vi "Link_Call Unlink.vi"(8 "error in (no error)":errorcluster, 11 "Run Data in":T1={"Target Folder"=path "", "Menu Folder"=path "", "Active Folder"=path "", "Config"={"Main"={"Menu Folder"="", "Re-Create Menu Folder?"=FALSE, "Allow mnu replace?"=FALSE, "Relative Link Target"="", "Auto Link?"=FALSE}, "File Filter"={"Exclude Prefixes"=[], "Ignore Names"=[], "Include Extensions"=[], "Exclude Postfixes"=[]}, "Folder Filter"={"Exclude Prefixes"=[], "Ignore Names"=[]}, "File Name Edit"={"Pre Split String"="", "Post Split String"="", "Deletion Strings"=[]}, "Folder Name Edit"={"Pre Split String"="", "Post Split String"="", "Deletion Strings"=[]}, "Folder Icon Map"={}, "Default Palette Data"={"Display Name Override"="", "View Format"=2, "Palette Width"=0, "Help Tag"="", "Help File Path"=path "", "Palette Description"=""}, "Default File Data"={"Display Name Override"="", "Place VI Contents?"=FALSE}, "Palette Override map"={}, "File Override map"={}}} {"Config"."Default Palette Data"."View Format" items=["Icons", "Text", "Icons and Text"]}) -> (0 "error out":errorcluster, 3 "Run Data out":T1={"Target Folder"=path "", "Menu Folder"=path "", "Active Folder"=path "", "Config"={"Main"={"Menu Folder"="", "Re-Create Menu Folder?"=FALSE, "Allow mnu replace?"=FALSE, "Relative Link Target"="", "Auto Link?"=FALSE}, "File Filter"={"Exclude Prefixes"=[], "Ignore Names"=[], "Include Extensions"=[], "Exclude Postfixes"=[]}, "Folder Filter"={"Exclude Prefixes"=[], "Ignore Names"=[]}, "File Name Edit"={"Pre Split String"="", "Post Split String"="", "Deletion Strings"=[]}, "Folder Name Edit"={"Pre Split String"="", "Post Split String"="", "Deletion Strings"=[]}, "Folder Icon Map"={}, "Default Palette Data"={"Display Name Override"="", "View Format"=2, "Palette Width"=0, "Help Tag"="", "Help File Path"=path "", "Palette Description"=""}, "Default File Data"={"Display Name Override"="", "Place VI Contents?"=FALSE}, "Palette Override map"={}, "File Override map"={}}} {"Config"."Default Palette Data"."View Format" items=["Icons", "Text", "Icons and Text"]})   [LabVIEW 2019, in "AutoMenuCreator.lvlib"]
uses:
  Ctl/Ctl_Run Data.ctl
  Ctl/Ctl_Config.ctl
  Ctl/Ctl_Config_Main.ctl
  Ctl/Ctl_Config_File Filter.ctl
  Ctl/Ctl_Config_Folder Filter.ctl
  Ctl/Ctl_Config_Name Edit.ctl
  Ctl/Ctl_Config_Folder Icon Map.ctl
  Ctl/Ctl_Config_Palette Data.ctl
  <vilib>/Palette API/Palette Menu/Public Type Define/View Format.ctl
  Ctl/Ctl_Config_File Data.ctl
  AutoMenuCreator.lvlib
  <vilib>/Palette API/Palette Menu/Palette Menu.lvlib
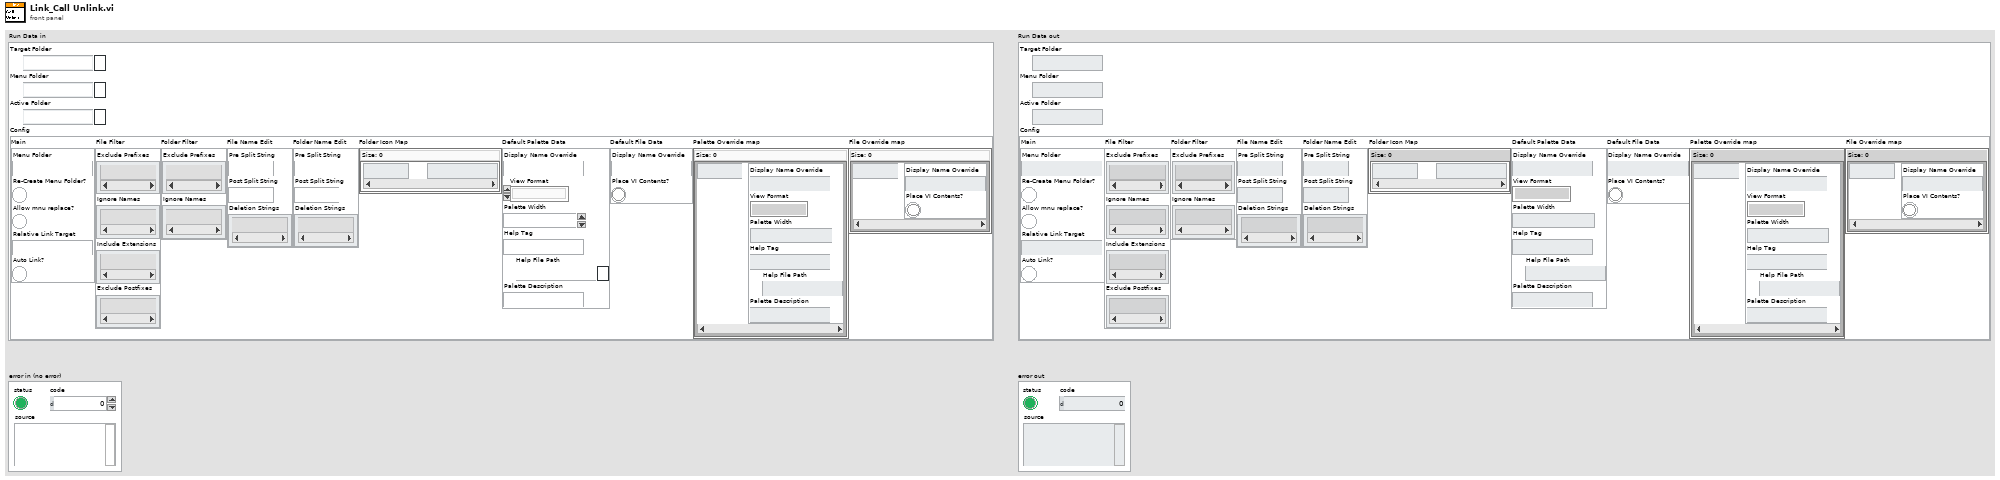
[diagram p1: front panel]
types:
  T1 = typedef "AutoMenuCreator.lvlib/Ctl_Run Data.ctl" = cluster{"Target Folder":path, "Menu Folder":path, "Active Folder":path, "Config":T2}
  T2 = typedef "AutoMenuCreator.lvlib/Ctl_Config.ctl" = cluster{"Main":T3, "File Filter":T4, "Folder Filter":T5, "File Name Edit":T6, "Folder Name Edit":T6, "Folder Icon Map":T7, "Default Palette Data":T8, "Default File Data":T10, "Palette Override map":map{string, T8}, "File Override map":map{string, T10}}
  T3 = typedef "AutoMenuCreator.lvlib/Ctl_Config_Main.ctl" = cluster{"Menu Folder":string, "Re-Create Menu Folder?":bool, "Allow mnu replace?":bool, "Relative Link Target":string, "Auto Link?":bool}
  T4 = typedef "AutoMenuCreator.lvlib/Ctl_Config_File Filter.ctl" = cluster{"Exclude Prefixes":string[], "Ignore Names":string[], "Include Extensions":string[], "Exclude Postfixes":string[]}
  T5 = typedef "AutoMenuCreator.lvlib/Ctl_Config_Folder Filter.ctl" = cluster{"Exclude Prefixes":string[], "Ignore Names":string[]}
  T6 = typedef "AutoMenuCreator.lvlib/Ctl_Config_Name Edit.ctl" = cluster{"Pre Split String":string, "Post Split String":string, "Deletion Strings":string[]}
  T7 = typedef "AutoMenuCreator.lvlib/Ctl_Config_Folder Icon Map.ctl" = map{string, path}
  T8 = typedef "AutoMenuCreator.lvlib/Ctl_Config_Palette Data.ctl" = cluster{"Display Name Override":string, "View Format":T9, "Palette Width":i16, "Help Tag":string, "Help File Path":path, "Palette Description":string}
  T9 = typedef "Palette Menu.lvlib/View Format.ctl" = u16
  T10 = typedef "AutoMenuCreator.lvlib/Ctl_Config_File Data.ctl" = cluster{"Display Name Override":string, "Place VI Contents?":bool}
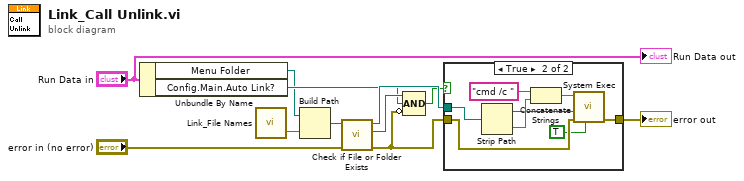
[diagram p0: block diagram]
diagram:
  n1 = Unbundle By Name("Run Data in") -> ("Menu Folder"=w1:path, "Config.Main.Auto Link?"=w5:bool)
  n2 = call "Link_File Names.vi"() -> ("Unlink file name"=w4:string)  [unwired: 2 in, 1 out]
  n3 = Build Path(base path=w1, name or relative path=w4) -> (appended path=w7:path)
  n4 = call <vilib>:"Check if File or Folder Exists.vi"("error in (no error)"="error in (no error)", "path"=w7) -> ("error out"=w8:errorcluster, "file or folder exists?"=w10:bool, "dup path"=w11:path)  [unwired: 7 in]
  n5 = Compound Arithmetic op=AND(w10, w5, invert w8) -> (w9:bool)
  n6 = case shown="True" w9 {
    tunnel: w11 -> [_ w16]
    tunnel: [w12 w14] -> w3
    tunnel: w8 -> [w12 w15]
    frame False {
    }
    frame True {
      n7 = Strip Path(path=w16) -> (stripped path=w18:path, name=w19:string)
      n8 = Concatenate Strings("cmd /c " ("string"), w19) -> (w17:string)
      n9 = call <vilib>:"System Exec.vi"("run minimized? (F)"=TRUE, "error in (no error)"=w15, "working directory"=w18, "command line"=w17) -> ("error out"=w14:errorcluster)  [unwired: 4 in, 3 out]
    }
  }
  "error out" <- w3
  "Run Data out" <- "Run Data in"
